vi "niFpgaPID_PIDMemoryRead.vi"(1 "channel (0)":u8) -> (4 "memory out":refnum<k21>="Data", 14 "parameters out":T1, 15 "state out":T2)   [LabVIEW 2017]
uses:
  <vilib>/rvi/Analysis/control/PID/Typedef/niFpgaPID_PIDState.ctl
  <vilib>/rvi/Analysis/control/PID/Typedef/niFpgaPID_PIDParameters.ctl
  <vilib>/Platform/TimedLoop/XDataNode/timing_clust.ctl
  <vilib>/Platform/TimedLoop/XDataNode/nitl_modes.ctl
  <vilib>/Platform/TimedLoop/XDataNode/wakeup.ctl
  <vilib>/rvi/Emulation/niFpgaSctlEmulationGetInTimedLoop.vi
  <vilib>/Utility/error.llb/Clear Errors.vi
  <vilib>/rvi/DataTransferAndStorage/Container/Common/niFpgaContainerGetUniqueNameForEmu.vi
  <vilib>/rvi/DataTransferAndStorage/Container/Common/niFpgaContainerSetEmuInfo.vi
  <vilib>/rvi/eio/common/nirviEmuReportErrorAndStop.vi
  <vilib>/rvi/DataTransferAndStorage/Container/Common/niFpgaContainerExecOnDevCompGetState.vi
  <vilib>/rvi/Emulation/niFpgaEmulationIsFPGAContextNoSignature.vi
  <vilib>/rvi/Emulation/niFpgaProcessEmulError.vi
  <vilib>/rvi/errors/nirviReportUnexpectedCaseInternalError (U32).vi
  <vilib>/rvi/Memory/Memory_Emulation/niFpgaMemoryEmulationCacheClearOnFirstRun.vi
  <vilib>/rvi/Memory/Memory_Emulation/nirvimemoryEmulationManagerCache_MakeExclusive.vi
  <vilib>/rvi/Memory/Memory_Emulation/niFpgaMemoryEmulationValidateCache.vi
  <vilib>/rvi/Memory/Memory_Emulation/nirvimemoryEmulationManagerCache_InsertValue.vi
  <vilib>/rvi/Memory/Memory_Emulation/nirvimemoryEmulationManagerCache_ReleaseExclusive.vi
  <vilib>/rvi/Memory/Memory_Emulation/nirvimemoryEmulationManagerCache_GetValue.vi
  <vilib>/rvi/Memory/Memory_Emulation/nirvimemoryEmulationManagerCache_SetValue.vi
  <vilib>/rvi/Emulation/niFpgaSctlEmulationResourceMgr.vi
  <vilib>/Platform/TimedLoop/XDataNode/XDataNode.xnode
  <vilib>/rvi/LocalResourceManager/LocalResourceManager.xnode
  <vilib>/rvi/DataTransferAndStorage/Container/XNode/niFpgaContainer.xnode
  <vilib>/rvi/Memory/Memory_Emulation/niFpgaMemoryEmulationRefIn.vi
  <vilib>/Platform/TimedLoop/XDataNode/XDNodeRunTimeDep.lvlib
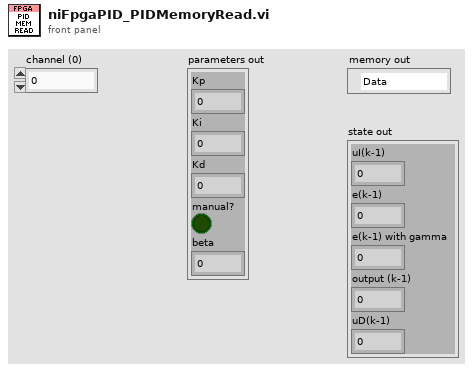
[diagram p1: front panel]
types:
  T1 = typedef "niFpgaPID_PIDParameters.ctl" = cluster{"Kp":sgl, "Ki":sgl, "Kd":sgl, "manual?":bool, "beta":sgl}
  T2 = typedef "niFpgaPID_PIDState.ctl" = cluster{"uI(k-1)":sgl, "e(k-1)":sgl, "e(k-1) with gamma":sgl, "output (k-1)":sgl, "uD(k-1)":sgl}
  T3 = typedef "XDNodeRunTimeDep.lvlib/timing_clust.ctl" = cluster{"Expected End [f-1]":u64, "Actual End [f-1]":u64, "Finished Late? [f-1]":bool, "Expected End [i-1]":u64, "Actual End [i-1]":u64, "Finished Late? [i-1]":bool, "Expected Start [i]":u64, "Actual Start [i]":u64, "Expected Start [f]":u64, "Actual Start [f]":u64, "Source Name":string, "Structure Name":string, "Period":i64, "Deadline":i64, "Offset":i64, "Start":i64, "Priority":i32, "Timeout":i32, "Mode":T4, "Wakeup Reason":T5, "Error":errorcluster, "Source Type":string, "Secondary Source Type":string, "Global End Time":u64, "Global Start Time":u64, "Frame Duration":u64, "Iteration Duration":u64, "Assigned CPU":i32, "I/O Scan Engine Mode":u32}
  T4 = typedef "XDNodeRunTimeDep.lvlib/nitl_modes.ctl" = enum32{"No Change", "Process missed periods, maintain original phase", "Discard missed periods, maintain original phase", "Process missed periods, ignore original phase", "Discard missed periods, ignore original phase"}
  T5 = typedef "XDNodeRunTimeDep.lvlib/wakeup.ctl" = enum32{"Normal", "Aborted", "Asynchronous wakeup", "Timing source error", "Timed loop error", "Timeout"}
  T6 = cluster{"data 1":sgl, "data 2":sgl, "data 3":sgl, "data 4":sgl, "data 5":sgl}
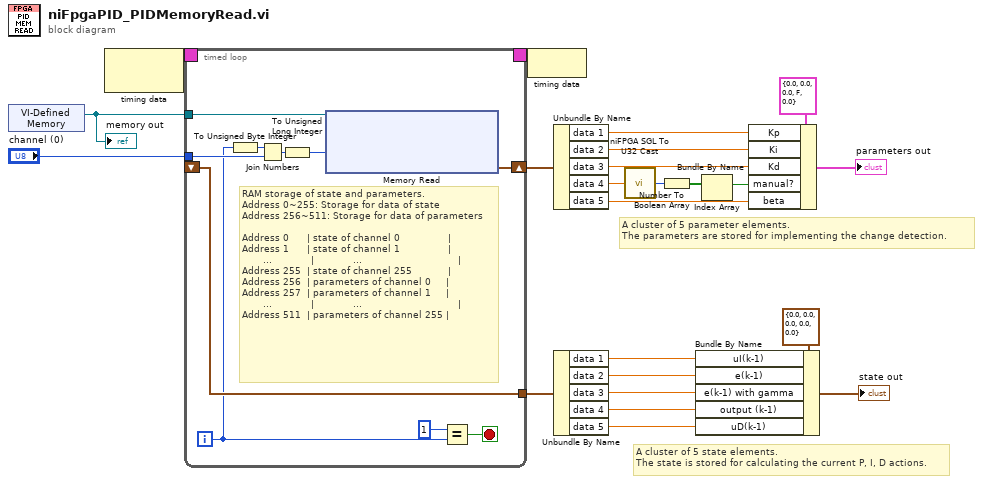
[diagram p0: block diagram]
diagram:
  # "A cluster of 5 parameter elements.\nThe parameters are stored for implementing the change detection."
  # "A cluster of 5 state elements.\nThe state is stored for calculating the current P, I, D actions."
  n1 = xnode "VI-Defined Memory"() -> ("Memory Out"=w20:refnum<k21>)
  "memory out" <- w20
  n2 = node-c288() -> (w23:T3)  [unwired: 1 in]
  n3 = timed-loop {
    tunnel: "channel (0)" -> [w30]
    timing: w23 -> [_]
    timing-out: [_] -> w22
    tunnel: w20 -> [w33]
    shift-right: [w32] -> w13
    shift-left: _ -> [w31]
    tunnel: [w31] -> w12
    i -> [w26]
    stop <- w28 stop-if-true
    # "RAM storage of state and parameters. \nAddress 0~255: Storage for data of state\nAddress 256~511: Storage for data of parameters\n                                                                         \nAddress 0      | state of channel 0                | \nAddress 1      | state of channel 1                | \n       ...             |             ...                                |\nAddress 255  | state of channel 255            | \nAddress 256  | parameters of channel 0     | \nAddress 257  | parameters of channel 1     | \n       ...             |             ...                                |\nAddress 511  | parameters of channel 255 |"
    n4 = To Unsigned Byte Integer(number=w26) -> (unsigned 8bit integer=w25:u8)
    n5 = Join Numbers(hi=w25, lo=w30) -> ((hi.lo)=w29:u16)
    n6 = To Unsigned Long Integer(number=w29) -> (unsigned 32bit integer=w27:u32)
    n7 = xnode "Memory Read"("Address"=w27, "Memory In"=w33) -> ("Data"=w32:T6)  [unwired: 1 out]
    n8 = Equal?(x=1, y=w26) -> (x = y?=w28:bool)
  }
  n9 = node-c288(w22) -> ()
  n10 = Unbundle By Name(w13) -> ("data 1"=w11:sgl, "data 2"=w10:sgl, "data 3"=w9:sgl, "data 4"=w8:sgl, "data 5"=w6:sgl)
  n11 = Unbundle By Name(w12) -> ("data 1"=w1:sgl, "data 2"=w2:sgl, "data 3"=w3:sgl, "data 4"=w4:sgl, "data 5"=w5:sgl)
  n12 = call <vilib>:"niFPGA SGL To U32 Cast.vi"("x"=w8) -> ("y"=w7:u32)  [unwired: 4 in]
  n13 = Number To Boolean Array(number=w7) -> (Boolean array=w15:bool[])
  n14 = Bundle By Name(cluster=T2 {"uI(k-1)"=0.0, "e(k-1)"=0.0, "e(k-1) with gamma"=0.0, "output (k-1)"=0.0, "uD(k-1)"=0.0} ("state out"), "uI(k-1)"=w1, "e(k-1)"=w2, "e(k-1) with gamma"=w3, "output (k-1)"=w4, "uD(k-1)"=w5) -> (→"state out":T2)
  n15 = Index Array(array=w15) -> (element=w14:bool)  [unwired: 1 in]
  n16 = Bundle By Name(cluster=T1 {"Kp"=0.0, "Ki"=0.0, "Kd"=0.0, "manual?"=FALSE, "beta"=0.0} ("parameters out"), "Kp"=w11, "Ki"=w10, "Kd"=w9, "manual?"=w14, "beta"=w6) -> (→"parameters out":T1)
